vi "checkStatus.vi"(8 "error in (no error)":errorcluster, 10 "stop":bool, 11 "ProEM_WinX32 in":refnum<class "ProEM_WinX32.lvclass">) -> (0 "error out":errorcluster, 2 "stopped?":bool, 3 "ProEM_WinX32 out":refnum<class "ProEM_WinX32.lvclass">)   [LabVIEW 2011, in "Hardware.lvlib" / "Channels.lvlib" / "ProEM_WinX32.lvclass"]
uses:
  ProEM_WinX32.lvclass
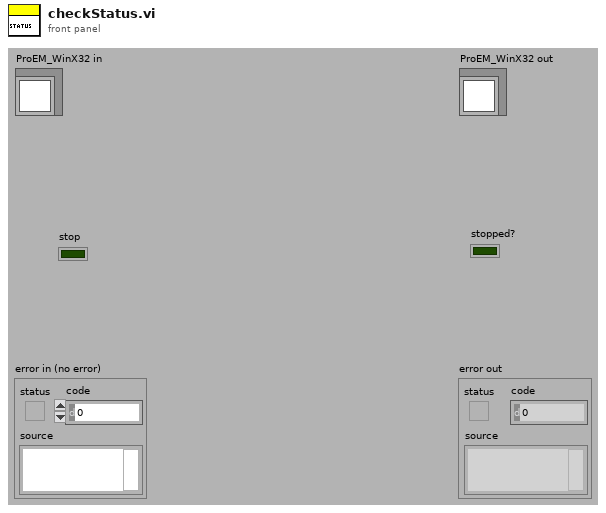
[diagram p1: front panel]
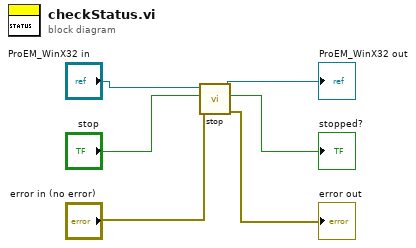
[diagram p0: block diagram]
diagram:
  n1 = call-dynamic "stop.vi"("error in (no error)"="error in (no error)", "stop"="stop", "ProEM_WinX32 in"="ProEM_WinX32 in") -> ("error out"=→"error out":errorcluster, "stopped?"=→"stopped?":bool, "ProEM_WinX32 out"=→"ProEM_WinX32 out":refnum<class "ProEM_WinX32.lvclass">)  [unwired: 5 in, 1 out]
